vi "create_application.vi"(5 "build_spec_name":string, 7 "build_artifact":path, 8 "error in (no error)":errorcluster, 10 "l3_zip_file_path":path, 11 "distribution_folder":path) -> (0 "error out":errorcluster)   [LabVIEW 2015, in "lv-builder-l3.lvlib"]
uses:
  lv-builder-l3.lvlib
  <userlib>/antonio-alexander/lv-bin-7zip/public/api/v1/_controls/config_value.ctl
  <userlib>/antonio-alexander/lv-bin-7zip/public/api/v1/_controls/config_include.ctl
  <userlib>/antonio-alexander/lv-bin-7zip/public/api/v1/advanced/extract_exe_archive.vi
  public/_subvis/advanced/create_batch-default.vi
  <userlib>/antonio-alexander/lv-bin-7zip/public/api/v1/advanced/compress_exe.vi
  <userlib>/antonio-alexander/lv-bin-7zip/public/api/v1/advanced/make_installer_exe_custom.vi
  <userlib>/antonio-alexander/lv-bin-7zip/public/api/v1/v1.lvlib
  <userlib>/antonio-alexander/lv-bin/public/api/v1/v1.lvlib
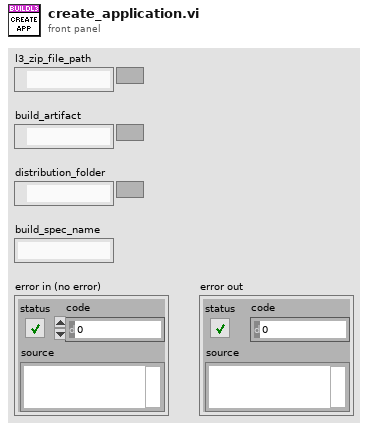
[diagram p1: front panel]
types:
  T1 = typedef "lv-bin-7zip.lvlib/v1.lvlib/config_include.ctl" = cluster{"title":bool, "begin_prompt":bool, "progress":bool, "run_program":bool, "directory":bool, "execute_file":bool, "execute_parameters":bool}
  T2 = typedef "lv-bin-7zip.lvlib/v1.lvlib/config_value.ctl" = cluster{"title":string, "begin_prompt":string, "run_program":string, "directory":string, "execute_file":string, "execute_parameters":string, "progress":bool}
  T3 = typedef "lv-bin.lvlib/v1.lvlib/temp_dir_config.ctl" = cluster{"root_folder":path, "prefix":string}
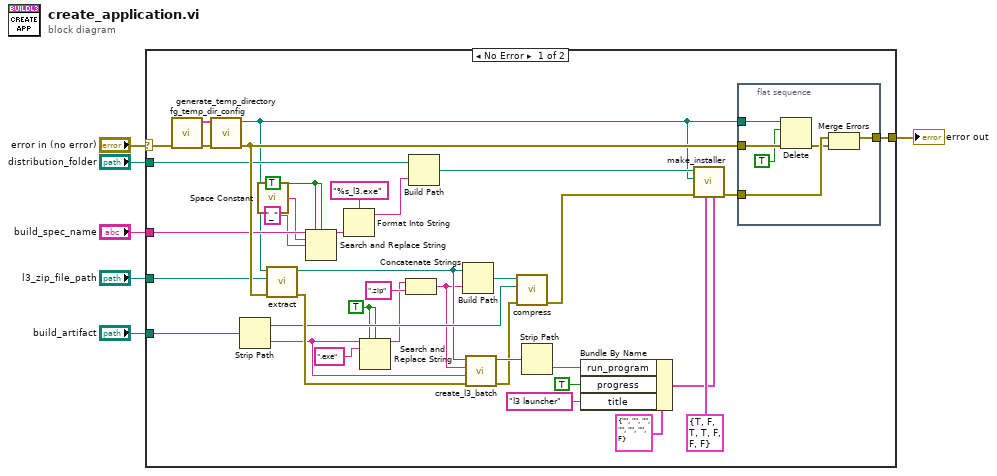
[diagram p0: block diagram]
diagram:
  n1 = case shown="No Error" "error in (no error)" {
    selector: "error in (no error)" -> [w18 w50]
    tunnel: "build_artifact" -> [w40 _]
    tunnel: "build_spec_name" -> [w39 _]
    tunnel: "distribution_folder" -> [w38 _]
    tunnel: [w37 w50] -> w3
    tunnel: "l3_zip_file_path" -> [w31 _]
    frame No Error {
      w15 = TRUE ("replace all? (F)")
      w24 = TRUE ("replace all? (F)")
      n2 = call "fg_temp_dir_config.vi"("error in (no error)"=w18) -> ("error out"=w30:errorcluster, "temp_dir_config out"=w29:T3)  [unwired: 9 in]
      n3 = call <userlib>:"generate_temp_directory.vi"("error in (no error)"=w30, "configuration"=w29) -> ("error out"=w42:errorcluster, "temp_dir"=w9:path)  [unwired: 8 in]
      n4 = Strip Path(path=w40) -> (stripped path=w41:path, name=w14:string)
      n5 = call <vilib>:"Space Constant.vi"() -> ("String"=w25:string)
      n6 = call-poly <userlib>:"extract.vi"("error in (no error)"=w42, "archive_path"=w31, "target_path in"=w9) -> ("error out"=w43:errorcluster, "target_path out"=w17:path)  [unwired: 5 in, 2 out]
      n7 = Search and Replace String(replace all?=w24, case sensitive?=w24, input string=w39, search string=w25, replace string="_" ("search string")) -> (result string=w27:string)  [unwired: 3 in, 3 out]
      n8 = Format Into String(format string="%s_l3.exe", w27) -> (resulting string=w20:string)  [unwired: 2 in, 1 out]
      n9 = Search and Replace String(replace all?=w15, case sensitive?=w15, input string=w14, search string=".exe") -> (result string=w13:string)  [unwired: 4 in, 3 out]
      n10 = Concatenate Strings(w13, ".zip" ("format string")) -> (w12:string)
      n11 = Build Path(base path=w38, name or relative path=w20) -> (appended path=w21:path)
      n12 = Build Path(base path=w17, name or relative path=w12) -> (appended path=w35:path)
      n13 = call-poly "create_l3_batch.vi"("error in (no error)"=w43, "application_command"=w14, "application_zip"=w12, "target_directory"=w17) -> ("error out"=w11:errorcluster, "batch_file"=w32:path)  [unwired: 6 in]
      n14 = call-poly <userlib>:"compress.vi"("error in (no error)"=w11, "files_to_add"=w41, "archive_path in"=w35) -> ("error out"=w10:errorcluster)  [unwired: 7 in, 1 out]
      n15 = Strip Path(path=w32) -> (name=w33:string)  [unwired: 1 out]
      n16 = Bundle By Name(cluster=T2 {"title"="", "begin_prompt"="", "run_program"="", "directory"="", "execute_file"="", "execute_parameters"="", "progress"=FALSE} ("config_value"), "run_program"=w33, "progress"=TRUE ("title"), "title"="l3 launcher") -> (w23:T2)
      n17 = call-poly <userlib>:"make_installer.vi"("config_value"=w23, "config_include"=T1 {"title"=TRUE, "begin_prompt"=FALSE, "progress"=TRUE, "run_program"=TRUE, "directory"=FALSE, "execute_file"=FALSE, "execute_parameters"=FALSE}, "error in (no error)"=w10, "installer_directory"=w9, "setup_filename in"=w21) -> ("error out"=w36:errorcluster)  [unwired: 5 in, 1 out]
      n18 = flat-sequence {
        tunnel: w9 -> [w49]
        tunnel: [w48] -> w37
        tunnel: w36 -> [w47]
        tunnel: w42 -> [w45]
        frame #0 {
          n19 = Delete(path (use dialog)=w49, entire hierarchy (F)=TRUE, error in=w45) -> (error out=w46:errorcluster)  [unwired: 2 in, 2 out]
          n20 = Merge Errors(w47, w46) -> (w48:errorcluster)
        }
      }
    }
    frame Error {
    }
  }
  "error out" <- w3
